vi "OpenShortDeEmbed_Write.vi"() -> ()   [LabVIEW 2017]
panel:
  out "error out":errorcluster
  in  "error in (no error)":errorcluster
  out "Intrinsic DUT S-parameter Trace Array":T1(array[cluster])=[{"Freq (Hz)"=5000000.0, "S-parameter Array"=[[0.0+0.0i, 1.0+0.0i], [1.0+0.0i, 0.0+0.0i]]}] {"Freq (Hz)" format="%.2e"; "S-parameter Array" format="%.3f"}
  in  "Short S-parameter File":path
  in  "Open S-parameter File":path
  in  "Extrinsic S-parameter File":path
  # "Performs Open-Short De-Embedding on 'extrinsic' S-parameters and Writes Result File\n\nAppends _OSdeembed to filename and puts in same folder"
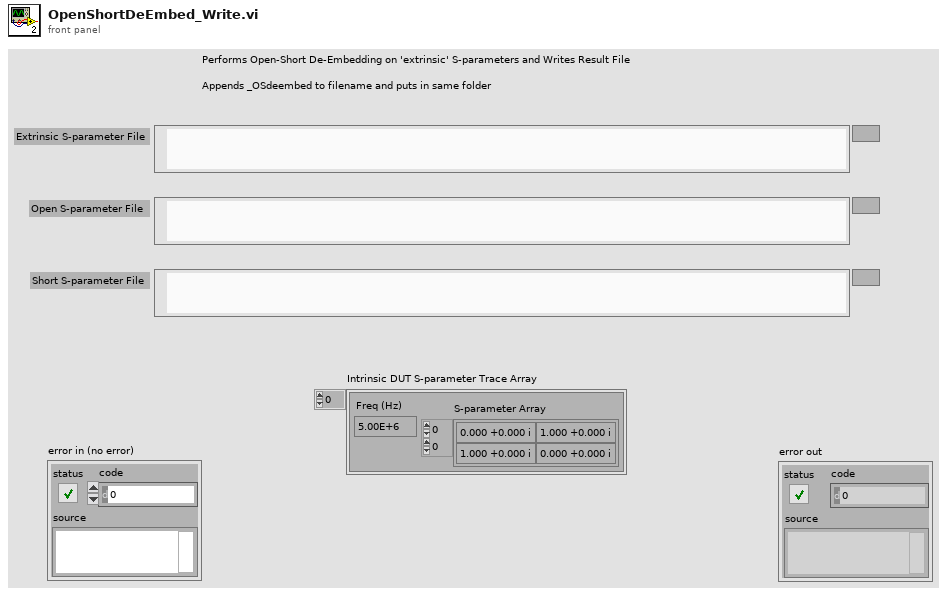
[diagram p1: front panel]
types:
  T1 = cluster{"Freq (Hz)":dbl, "S-parameter Array":csg[][]}[]
  T2 = cluster{"Comments":string, "Ref Impedance":u16, "Trace Array":cluster{"Freq (Hz)":dbl, "S-parameter Array":cdb[][]}[]}
  T3 = cluster{"Freq (Hz)":dbl, "S-parameter Array":cdb[][]}[]
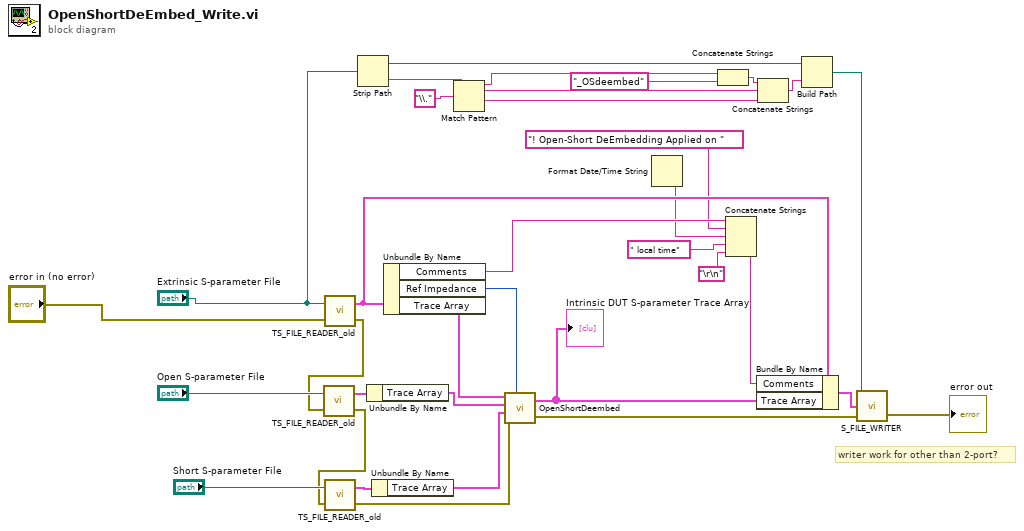
[diagram p0: block diagram]
diagram:
  # "writer work for other than 2-port?"
  n1 = call "TS_FILE_READER_old.VI"("error in (no error)"="error in (no error)", "File"="Extrinsic S-parameter File") -> ("error out"=w32:errorcluster, "Data Output"=w20:T2)
  n2 = call "TS_FILE_READER_old.VI"("error in (no error)"=w32, "File"="Open S-parameter File") -> ("error out"=w31:errorcluster, "Data Output"=w29:T2)
  n3 = call "TS_FILE_READER_old.VI"("error in (no error)"=w31, "File"="Short S-parameter File") -> ("error out"=w25:errorcluster, "Data Output"=w30:T2)
  n4 = Strip Path(path="Extrinsic S-parameter File") -> (stripped path=w10:path, name=w8:string)
  n5 = Unbundle By Name(w29) -> ("Trace Array"=w27:T3)
  n6 = Unbundle By Name(w30) -> ("Trace Array"=w26:T3)
  n7 = Unbundle By Name(w20) -> ("Comments"=w16:string, "Ref Impedance"=w24:u16, "Trace Array"=w28:T3)
  n8 = Match Pattern(string=w8, regular expression="\\.") -> (before substring=w2:string, match substring=w4:string, after substring=w5:string)  [unwired: 1 in, 1 out]
  n9 = call "OpenShortDeembed.vi"("Extrinsic DUT S-parameter Trace Array"=w28, "Open S-parameter Trace Array"=w27, "Short S-parameter Trace Array"=w26, "error in (no error)"=w25, "Reference Impedance"=w24) -> ("Intrinsic DUT S-parameter Trace Array"=w18:T1, "error out"=w22:errorcluster)
  "Intrinsic DUT S-parameter Trace Array" <- w18
  n10 = Format Date/Time String() -> (date/time string=w13:string)  [unwired: 3 in]
  n11 = Concatenate Strings(w2, "_OSdeembed") -> (w3:string)
  n12 = Concatenate Strings(w16, "! Open-Short DeEmbedding Applied on ", w13, " local time", "\r\n") -> (w19:string)
  n13 = Bundle By Name(cluster=w20, "Comments"=w19, "Trace Array"=w18) -> (w17:T2)
  n14 = Concatenate Strings(w3, w4, w5) -> (w6:string)
  n15 = Build Path(base path=w10, name or relative path=w6) -> (appended path=w9:path)
  n16 = call "S_FILE_WRITER.VI"("error in (no error)"=w22, "Data Input"=w17, "Input Path"=w9) -> ("error out"=→"error out":errorcluster)  [unwired: 1 in, 1 out]
